vi "PDO unlink.vi"(4 "Wait?":bool, 5 "error in (no error)":errorcluster, 6 "Indices":cluster{"Communication":u32, "Mapping":u32}={"Communication"=6144, "Mapping"=6656} {"Mapping" format="%x"; "Communication" format="%x"}, 7 "Cob ID":u32, 8 "CANopen in":refnum<class "CANopen.lvclass">) -> (0 "error out":errorcluster, 3 "CANopen out":refnum<class "CANopen.lvclass">)   [LabVIEW 2017, in "canopen.lvlib" / "CANopen.lvclass"]
doc: "Links a PDO COB-ID to a specific map of OD items."
uses:
  CANopen.lvclass
  SDO download (U8).vi
  SDO download (U32).vi
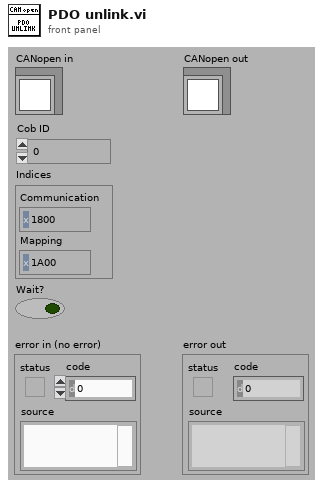
[diagram p1: front panel]
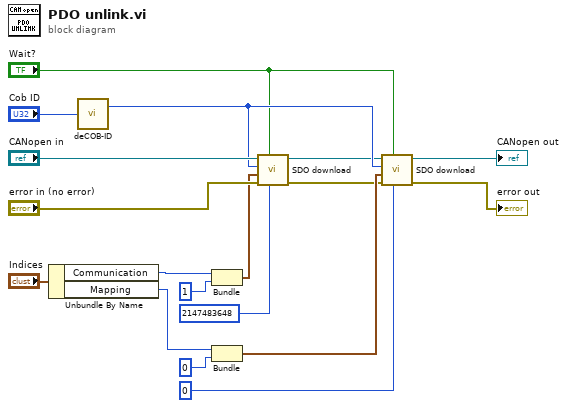
[diagram p0: block diagram]
diagram:
  n1 = Unbundle By Name("Indices") -> ("Communication"=w8:u32, "Mapping"=w9:u32)
  n2 = call "deCOB-ID.vi"("Cob ID"="Cob ID") -> ("Node ID"=w7:u16)  [unwired: 1 out]
  n3 = Bundle("Communication"=w8, "Sub-index"=u8 1) -> (w12:cluster{"Communication":u32, "Sub-index":u8})  [unwired: 1 out]
  n4 = Bundle("Mapping"=w9, "Sub-index"=u8 0) -> (w11:cluster{"Mapping":u32, "Sub-index":u8})  [unwired: 1 out]
  n5 = call-poly "SDO download.vi"("Value"=u32 2147483648 ("Communication index"), "Wait?"="Wait?", "error in (no error)"="error in (no error)", "Multiplexor"=w12, "Node ID"=w7, "CANopen in"="CANopen in") -> ("error out"=w4:errorcluster, "CANopen out"=w5:refnum<class "CANopen.lvclass">)  [unwired: 2 out]
  n6 = call-poly "SDO download.vi"("Value"=u8 0 ("Sub-index"), "Wait?"="Wait?", "error in (no error)"=w4, "Multiplexor"=w11, "Node ID"=w7, "CANopen in"=w5) -> ("error out"=→"error out":errorcluster, "CANopen out"=→"CANopen out":refnum<class "CANopen.lvclass">)  [unwired: 2 out]
